vi "host_get_data.vi"(8 "error in":errorcluster) -> (0 "error IO":errorcluster)   [LabVIEW 2021]
uses:
  host_global_vars.vi
  <vilib>/Utility/error.llb/Error Cluster From Error Code.vi
  <vilib>/rvi/errors/niLvFpgaAdjustHostInterfaceError.vi
  <vilib>/rvi/interface/nirviReadWriteControl/nirviReadWriteControl.xnode
  FPGA Bitfiles/openlabspm_FPGATarget_fpgamain_eo-gUZR5D1g.lvbitx
  fpga/fpga_main.vi
  NiFpgaLv.dll
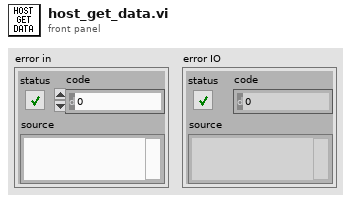
[diagram p1: front panel]
types:
  T1 = typedef "fpga_dtype_status.ctl" = cluster{"scanning":bool, "new target":bool, "move completed":bool, "measure completed":bool, "inrange":bool, "ready to move":bool, "output inrange":bool, "tip guard":bool}
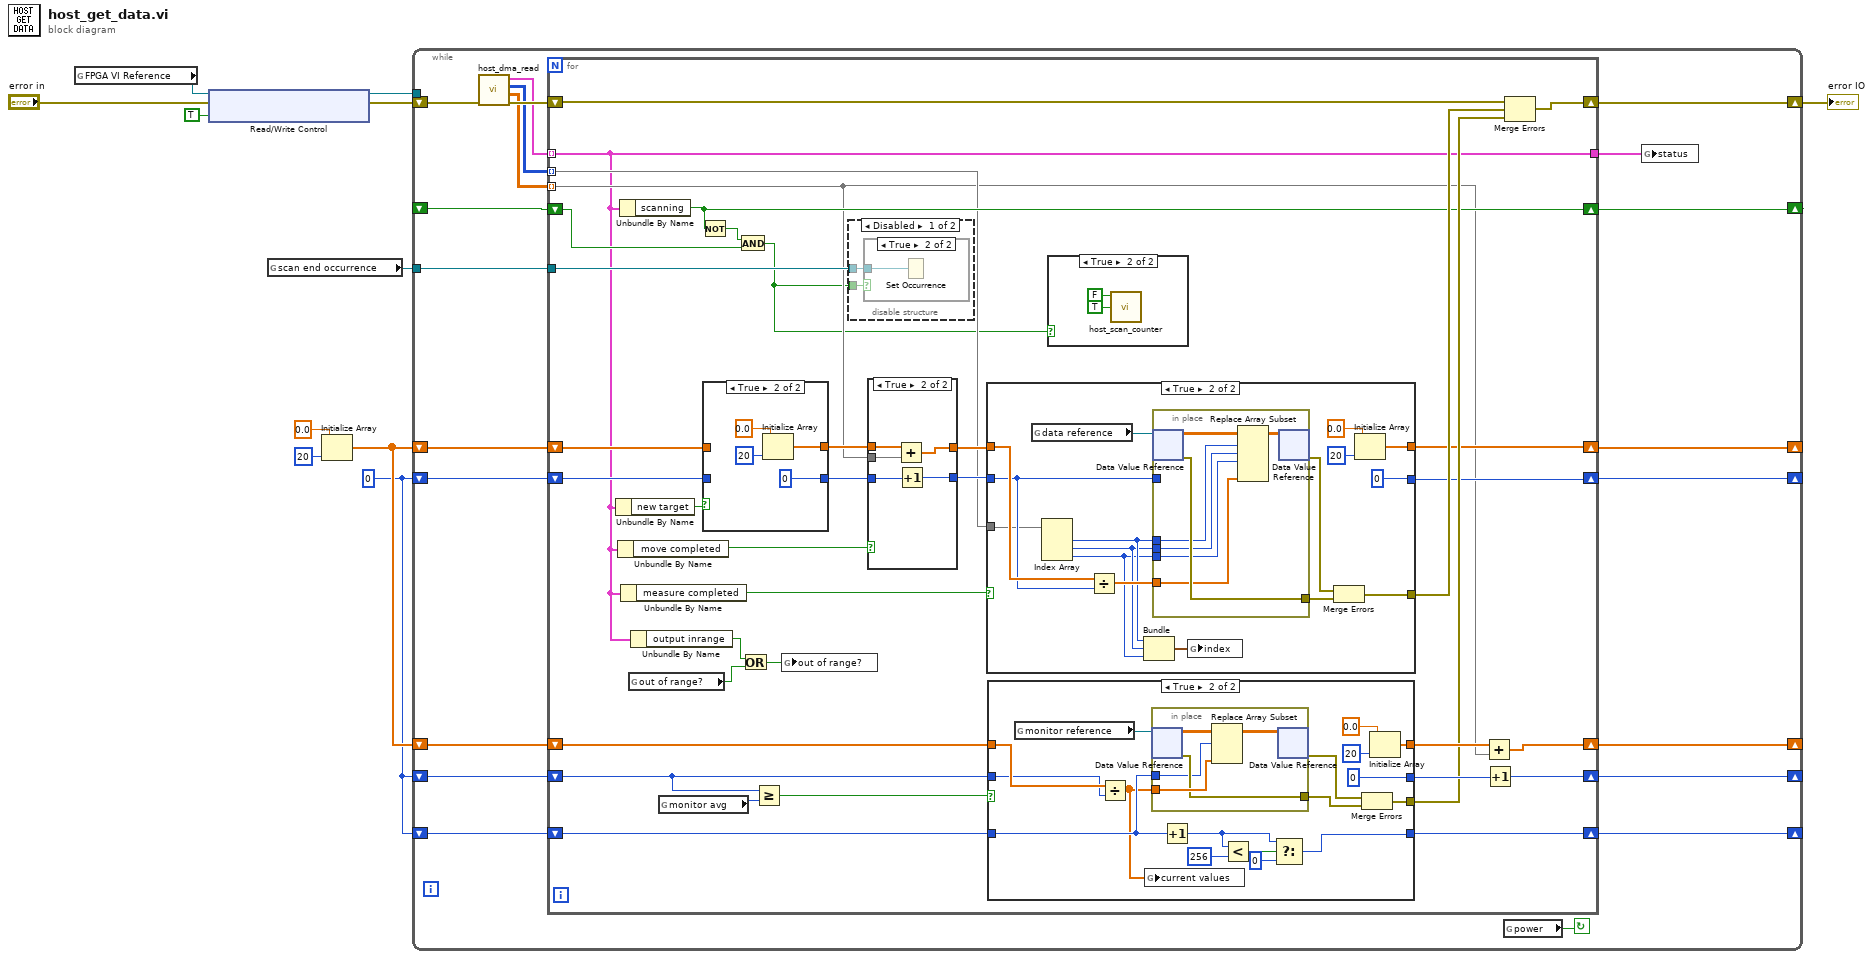
[diagram p0: block diagram]
diagram:
  w2 = 0
  n1 = global read "host_global_vars.vi" "FPGA VI Reference"() -> (w11:refnum<k20>)
  n2 = xnode "Read/Write Control"("FPGA VI Reference In"=w11, "error in"="error in", "DMA"=TRUE) -> ("FPGA VI Reference Out"=w10:refnum<k20>, "error out"=w8:errorcluster)
  n3 = global read "host_global_vars.vi" "scan end occurrence"() -> (w1:refnum<k4>)
  n4 = Initialize Array(sgl 0.0 ("element"), 20 ("dimension size")) -> (w4:sgl[])
  n5 = while {
    tunnel: w10 -> [_]
    shift-right: [w31] -> w3
    shift-left: w8 -> [w19]
    shift-right: [w26] -> _
    shift-left: w4 -> [w30]
    shift-right: [w23] -> _
    shift-left: w4 -> [w29]
    shift-right: [w25] -> _
    shift-left: w2 -> [w28]
    shift-right: [w24] -> _
    shift-left: w2 -> [w27]
    shift-right: [w21] -> _
    shift-left: w2 -> [w22]
    tunnel: w1 -> [w20]
    shift-right: [w14] -> _
    shift-left: _ -> [w13]
    stop <- w32 continue-if-true
    n6 = call "host_dma_read.vi"("error in"=w19) -> ("error out"=w18:errorcluster, "values"=w15:sgl[][], "indices"=w16:i16[][], "status"=w17:T1[])  [unwired: 7 in]
    n7 = for {
      shift-right: [w57] -> w31
      shift-left: w18 -> [w60]
      shift-right: [w68] -> w23
      shift-left: w29 -> [w63]
      shift-right: [w40] -> w26
      shift-left: w30 -> [w49]
      shift-right: [w41] -> w25
      shift-left: w28 -> [w48]
      shift-right: [w67] -> w24
      shift-left: w27 -> [w62]
      shift-right: [w55] -> w21
      shift-left: w22 -> [w56]
      tunnel: w20 -> [w54]
      tunnel: w17 -> [w37] mode=indexing
      tunnel: w16 -> [w39] mode=indexing
      tunnel: w15 -> [w38] mode=indexing
      shift-right: [w52] -> w14
      shift-left: w13 -> [w51]
      tunnel: [w37] -> w12
      n8 = Unbundle By Name(w37) -> ("new target"=w50:bool)
      n9 = Unbundle By Name(w37) -> ("move completed"=w47:bool)
      n10 = Unbundle By Name(w37) -> ("scanning"=w52:bool)
      n11 = Unbundle By Name(w37) -> ("measure completed"=w44:bool)
      n12 = global read "host_global_vars.vi" "out of range?"() -> (w35:bool)
      n13 = Unbundle By Name(w37) -> ("output inrange"=w36:bool)
      n14 = global read "host_global_vars.vi" "monitor avg"() -> (w64:i32)
      n15 = Not(x=w52) -> (.not. x?=w53:bool)
      n16 = case shown="True" w50 {
        tunnel: [w75 w77] -> w46
        tunnel: w49 -> [w75 _]
        tunnel: [w74 0] -> w45
        tunnel: w48 -> [w74 _]
        frame False {
        }
        frame True {
          n17 = Initialize Array(sgl 0.0 ("element"), 20 ("dimension size")) -> (w77:sgl[])
        }
      }
      n18 = And(x=w53, y=w51) -> (x .and. y?=w33:bool)
      n19 = Or(x=w36, y=w35) -> (x .or. y?=w34:bool)
      n20 = Greater Or Equal?(x=w62, y=w64) -> (x >= y?=w61:bool)
      n21 = global write "host_global_vars.vi" "out of range?"(w34) -> ()
      n22 = disable-structure shown="Disabled" {
        disable-tunnel: w54 -> [w72 _]
        disable-tunnel: w33 -> [w71 _]
        frame Disabled {
          n23 = case shown="True" w71 {
            tunnel: w72 -> [_ w73]
            frame False {
            }
            frame True {
              n24 = Set Occurrence(w73) -> ()
            }
          }
        }
        frame Enabled {
        }
      }
      n25 = case shown="True" w47 {
        tunnel: [w81 w86] -> w42
        tunnel: [w80 w85] -> w43
        tunnel: w46 -> [w81 w84]
        tunnel: w45 -> [w80 w83]
        tunnel: w38 -> [_ w82]
        frame False {
        }
        frame True {
          n26 = Add(x=w84, y=w82) -> (x+y=w86:sgl[])
          n27 = Increment(x=w83) -> (x+1=w85:i32)
        }
      }
      n28 = case shown="True" w44 {
        tunnel: [w87 w93] -> w40
        tunnel: [w88 0] -> w41
        tunnel: w42 -> [w87 w102]
        tunnel: w43 -> [w88 w101]
        tunnel: [_ w98] -> w59
        tunnel: w39 -> [_ w97]
        frame False {
        }
        frame True {
          n29 = global read "host_global_vars.vi" "data reference"() -> (w104:refnum<data-value>)
          n30 = Index Array(array=w97) -> (element #1=w91:i16, element #2=w90:i16, element #3=w89:i16)  [unwired: 3 in]
          n31 = Divide(x=w102, y=w101) -> (x/y=w103:sgl[])
          n32 = Bundle(w91, w90, w89) -> (w92:cluster{i16, i16, i16})  [unwired: 1 in]
          n33 = in-place {
            in-place-border: w101 -> [_]
            in-place-border: w103 -> [w105]
            in-place-border: [w109] -> w99
            in-place-border: w91 -> [w108]
            in-place-border: w90 -> [w107]
            in-place-border: w89 -> [w106]
            n34 = in-place-dvr #1(w104) -> (w111:sgl[][][][], w109:errorcluster)
            n35 = Replace Array Subset(array=w111, new element=w105, index (dim 0)=w108, index (dim 1)=w107, index (dim 2)=w106) -> (w110:sgl[][][][])  [unwired: 1 in]
            n36 = in-place-dvr #1(w110) -> (w100:errorcluster)  [unwired: 1 out]
          }
          n37 = global write "host_global_vars.vi" "index"(w92) -> ()
          n38 = Merge Errors(w100, w99) -> (w98:errorcluster)
          n39 = Initialize Array(sgl 0.0 ("element"), 20 ("dimension size")) -> (w93:sgl[])
        }
      }
      n40 = case shown="True" w61 {
        tunnel: [w113 w129] -> w66
        tunnel: [w114 0] -> w65
        tunnel: w63 -> [w113 w126]
        tunnel: w62 -> [w114 w125]
        tunnel: [_ w122] -> w58
        tunnel: w56 -> [w112 w121]
        tunnel: [w112 w116] -> w55
        frame False {
        }
        frame True {
          n41 = global read "host_global_vars.vi" "monitor reference"() -> (w127:refnum<data-value>)
          n42 = Divide(x=w126, y=w125) -> (x/y=w115:dbl[])
          n43 = global write "host_global_vars.vi" "current values"(w115) -> ()
          n44 = in-place {
            in-place-border: w115 -> [w135]
            in-place-border: [w133] -> w123
            in-place-border: w121 -> [w132]
            n45 = in-place-dvr #2(w127) -> (w136:sgl[][], w133:errorcluster)
            n46 = Replace Array Subset(array=w136, new element=w135, index (row)=w132) -> (w134:sgl[][])  [unwired: 1 in]
            n47 = in-place-dvr #2(w134) -> (w124:errorcluster)  [unwired: 1 out]
          }
          n48 = Increment(x=w121) -> (x+1=w118:i32)
          n49 = Less?(x=w118, y=256) -> (x < y?=w119:bool)
          n50 = Select(t=w118, s=w119, f=0) -> (s? t:f=w116:i32)
          n51 = Merge Errors(w124, w123) -> (w122:errorcluster)
          n52 = Initialize Array(0.0 ("element"), 20 ("dimension size")) -> (w129:dbl[])
        }
      }
      n53 = case shown="True" w33 {
        frame False {
        }
        frame True {
          n54 = call "host_scan_counter.vi"("update?"=TRUE, "count up?"=FALSE) -> ()  [unwired: 9 in, 1 out]
        }
      }
      n55 = Add(x=w66, y=w38) -> (x+y=w68:dbl[])
      n56 = Increment(x=w65) -> (x+1=w67:i32)
      n57 = Merge Errors(w60, w59, w58) -> (w57:errorcluster)
    }
    n58 = global read "host_global_vars.vi" "power"() -> (w32:bool)
    n59 = global write "host_global_vars.vi" "status"(w12) -> ()
  }
  "error IO" <- w3
